vi "Main.vi"() -> ()   [LabVIEW 2014]
doc: "Program główny. (Jak narazie)\nTime w kliencie można interpretować jako sekundy (nie jest to oczywiste, bo ma typ double)."
uses:
  Client.ctl
  Kasy.ctl
  LukiBrary.lvlib
panel:
  out "size(s)":i32
  out "Waveform Chart":i32(graph)
  out "# elements in queue":i32
  out "Obsługiwanych klientów":i32
  out "Kasa 2":T1
  in  "Max czas obsługi":dbl
  in  "Kasa":T1={"Zarobek"=0, "Liczba kas"=4, "Czas"=[]}
  out "People":T2[](array[typedef])
  in  "lambda":dbl=1.0 format="%#_13g"
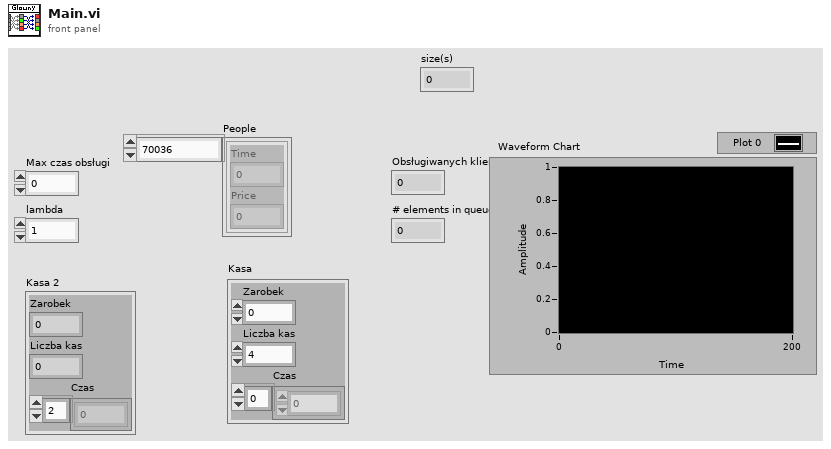
[diagram p1: front panel]
types:
  T1 = typedef "Kasy.ctl" = cluster{"Zarobek":i32, "Liczba kas":u8, "Czas":i32[]}
  T2 = typedef "LukiBrary.lvlib/Client.ctl" = cluster{"Time":i32, "Price":i32}
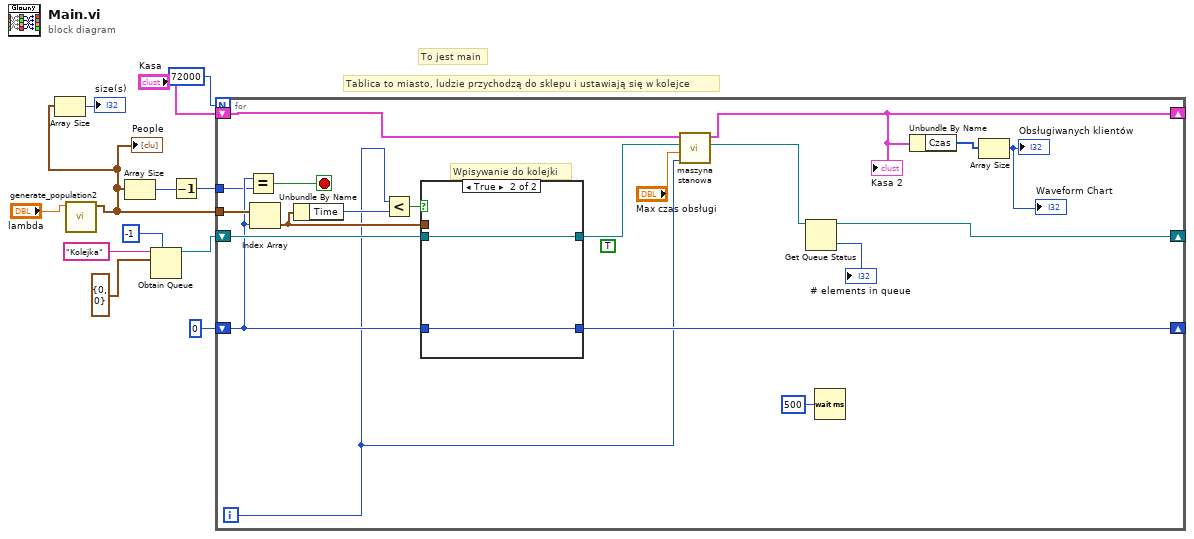
[diagram p0: block diagram]
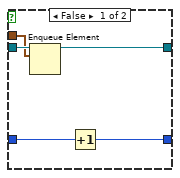
[diagram p2: hidden frame]
diagram:
  # "To jest main"
  # "Tablica to miasto, ludzie przychodzą do sklepu i ustawiają się w kolejce"
  n1 = call "generate_population2.vi"("lambda"="lambda") -> ("Array"=w2:T2[])  [unwired: 10 in]
  "People" <- w2
  n2 = Array Size(array=w2) -> (size(s)=→"size(s)":i32)
  n3 = Array Size(array=w2) -> (size(s)=w7:i32)
  n4 = Obtain Queue(max queue size (-1, unlimited)=-1, name (unnamed)="Kolejka", element data type=T2 {"Time"=0, "Price"=0} ("Client")) -> (queue out=w8:refnum<queue>)  [unwired: 2 in, 2 out]
  n5 = Decrement(x=w7) -> (x-1=w6:i32)
  n6 = for {
    N: 72000 -> [_]
    tunnel: w2 -> [w32]
    shift-right: [w28] -> _
    shift-left: 0 -> [w26]
    shift-right: [w18] -> _
    shift-left: w8 -> [w27]
    tunnel: w6 -> [w25]
    shift-right: [w20] -> _
    shift-left: "Kasa" -> [w24]
    i -> [w15]
    stop <- w14 stop-if-true
    (unwired) TRUE ("return elements? (F)")
    # "Wpisywanie do kolejki"
    n7 = Equal?(x=w26, y=w25) -> (x = y?=w14:bool)
    n8 = Index Array(array=w32, index=w26) -> (element=w29:T2)
    n9 = Unbundle By Name(w29) -> ("Time"=w31:i32)
    n10 = Less?(x=w15, y=w31) -> (x < y?=w30:bool)
    n11 = case shown="True" w30 {
      tunnel: w26 -> [w37 w39]
      tunnel: [w36 w39] -> w28
      tunnel: w29 -> [w33 _]
      tunnel: w27 -> [w35 w38]
      tunnel: [w34 w38] -> w22
      frame False {
        n12 = Enqueue Element(queue=w35, element=w33) -> (queue out=w34:refnum<queue>)  [unwired: 2 in, 2 out]
        n13 = Increment(x=w37) -> (x+1=w36:i32)
      }
      frame True {
      }
    }
    n14 = call "maszyna stanowa.vi"("Current Time"=w15, "Max czas obsługi"="Max czas obsługi", "Queue in"=w22, "Kasa"=w24) -> ("Queue in 2"=w21:refnum<queue>, "Kasa 2"=w20:T1)  [unwired: 6 in]
    "Kasa 2" <- w20
    n15 = Get Queue Status(queue=w21) -> (queue out=w18:refnum<queue>, # elements in queue=→"# elements in queue":i32)  [unwired: 2 in, 6 out]
    n16 = Wait (ms)(milliseconds to wait=u32 500) -> ()  [unwired: 1 out]
    n17 = Unbundle By Name(w20) -> ("Czas"=w19:i32[])
    n18 = Array Size(array=w19) -> (size(s)=→"Obsługiwanych klientów" →"Waveform Chart":i32)
  }
